vi "Configure LTI ULS.vi"(8 "error in (no error)":errorcluster, 10 "Datalogger Enqueuer":refnum<class "Message Enqueuer.lvclass">, 11 "LTI ULS Actor in":refnum<class "LTI ULS Actor.lvclass">) -> (0 "error out":errorcluster, 3 "LTI ULS Actor out":refnum<class "LTI ULS Actor.lvclass">)   [LabVIEW 2018, in "LTI ULS Actor.lvlib" / "LTI ULS Actor.lvclass"]
uses:
  LTI ULS Actor.lvclass
  C:/Users/dev/Documents/CODE/LabVIEW/microwaveverify/trunk/MWWL Verification/Sensor Actor/Sensor/Sensor.lvclass
  C:/Program Files (x86)/National Instruments/LabVIEW 2018/vi.lib/ActorFramework/Actor/Actor.lvclass
  <vilib>/ActorFramework/Message Enqueuer/Message Enqueuer.lvclass
  LTI ULS Actor.lvclass/LTI ULS Actor.ctl
  <vilib>/ActorFramework/Actor/Actor.lvclass/Actor.ctl
  MWWL Verification/MWWL Verification Messages/Log Event Msg/Log Event Msg.lvclass/Log Event Msg.ctl
  <vilib>/ActorFramework/Message Enqueuer/Message Enqueuer.lvclass/Message Enqueuer.ctl
  <vilib>/ActorFramework/Message Enqueuer/Enqueue.vi
  MWWL Verification/MWWL Verification Messages/Log Event Msg/Log Event Msg.lvclass
  C:/Program Files (x86)/National Instruments/LabVIEW 2018/vi.lib/ActorFramework/Message/Message.lvclass
  <vilib>/Instr/_visa.llb/VISA Configure Serial Port (Instr).vi
  <vilib>/ActorFramework/Message Priority Queue/Priority Enqueue.vi
  Sensor Actor/Sensor/Sensor.lvclass
  <vilib>/ActorFramework/Actor/Actor.lvclass
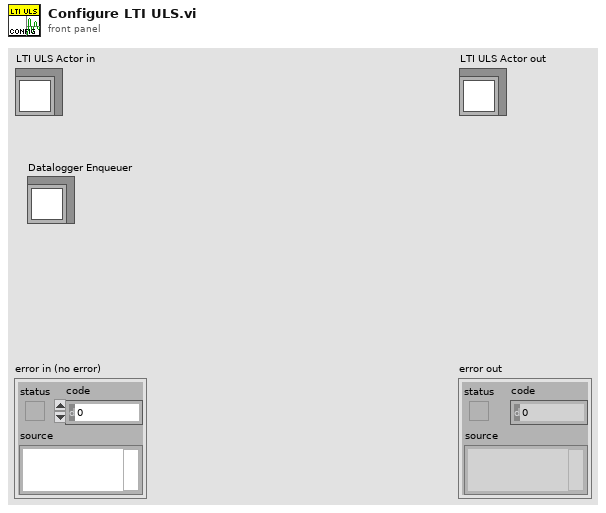
[diagram p1: front panel]
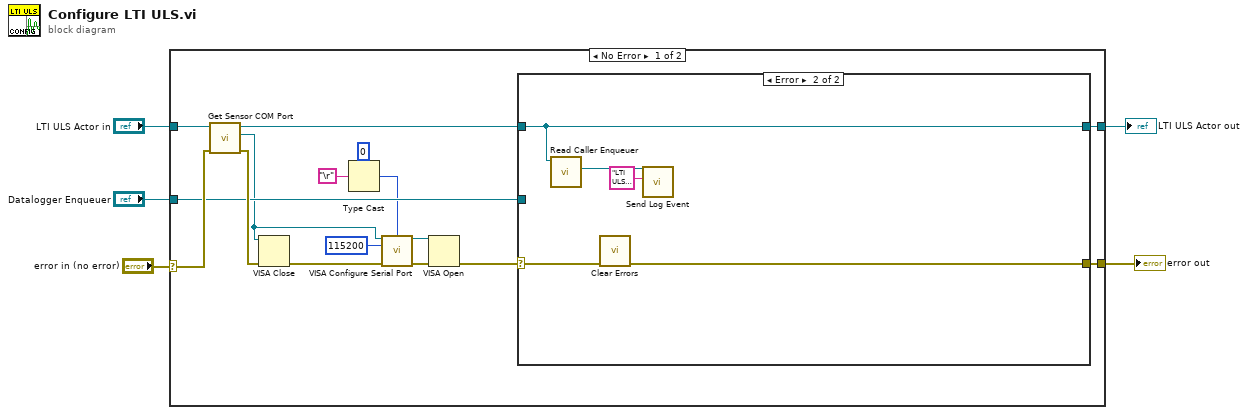
[diagram p0: block diagram]
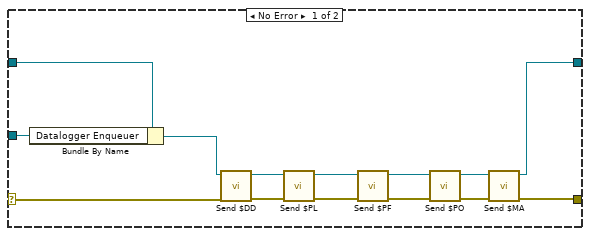
[diagram p2: hidden frame]
diagram:
  n1 = case shown="No Error" "error in (no error)" {
    selector: "error in (no error)" -> [w12 w42]
    tunnel: [w14 w42] -> w4
    tunnel: [w15 w41] -> w2
    tunnel: "LTI ULS Actor in" -> [w21 w41]
    tunnel: "Datalogger Enqueuer" -> [w11 _]
    frame No Error {
      n2 = call "Get Sensor COM Port.vi"("error in (no error)"=w12, "Sensor in"=w21) -> ("error out"=w13:errorcluster, "COM Port"=w9:refnum<visa-resource-name>, "Sensor out"=w16:refnum<class "LTI ULS Actor.lvclass">)  [unwired: 7 in]
      n3 = VISA Close(VISA resource name=w9, error in (no error)=w13) -> (error out=w20:errorcluster)
      n4 = Type Cast(type=u8 0 ("termination char\n(0xA = '\\n' = LF)"), x="\r") -> (*(type *) &x=w7:u8)
      n5 = call-poly "VISA Configure Serial Port"("VISA resource name"=w9, "termination char\n(0xA = '\\n' = LF)"=w7, "baud rate (9600)"=u32 115200, "error in (no error)"=w20) -> ("VISA resource name out"=w18:refnum<visa-resource-name>, "error out"=w19:errorcluster)  [unwired: 10 in]
      n6 = VISA Open(error in (no error)=w19, VISA resource name=w18) -> (error out=w17:errorcluster)  [unwired: 3 in, 1 out]
      n7 = case shown="Error" w17 {
        selector: w17 -> [w33 w38]
        tunnel: w16 -> [w34 w36]
        tunnel: [w25 w36] -> w15
        tunnel: [w26 w37] -> w14
        tunnel: w11 -> [w35 _]
        frame No Error {
          n8 = Bundle By Name(cluster=w34, "Datalogger Enqueuer"=w35) -> (w31:refnum<class "LTI ULS Actor.lvclass">)
          n9 = call "Send $DD.vi"("error in (no error)"=w33, "LTI ULS Actor in"=w31) -> ("error out"=w32:errorcluster, "LTI ULS Actor out"=w30:refnum<class "LTI ULS Actor.lvclass">)  [unwired: 8 in]
          n10 = call "Send $PL.vi"("error in (no error)"=w32, "LTI ULS Actor in"=w30) -> ("error out"=w29:errorcluster, "LTI ULS Actor out"=w22:refnum<class "LTI ULS Actor.lvclass">)  [unwired: 8 in]
          n11 = call "Send $PF.vi"("error in (no error)"=w29, "LTI ULS Actor in"=w22) -> ("error out"=w28:errorcluster, "LTI ULS Actor out"=w23:refnum<class "LTI ULS Actor.lvclass">)  [unwired: 8 in]
          n12 = call "Send $PO.vi"("error in (no error)"=w28, "LTI ULS Actor in"=w23) -> ("error out"=w27:errorcluster, "LTI ULS Actor out"=w24:refnum<class "LTI ULS Actor.lvclass">)  [unwired: 8 in]
          n13 = call "Send $MA.vi"("error in (no error)"=w27, "LTI ULS Actor in"=w24) -> ("error out"=w26:errorcluster, "LTI ULS Actor out"=w25:refnum<class "LTI ULS Actor.lvclass">)  [unwired: 8 in]
        }
        frame Error {
          n14 = call <vilib>:"Read Caller Enqueuer.vi"("Actor"=w36) -> ("Caller Enqueuer"=w40:refnum<class "Message Enqueuer.lvclass">)  [unwired: 10 in]
          n15 = call <vilib>:"Clear Errors.vi"("error in (no error)"=w38) -> ("error out"=w37:errorcluster)  [unwired: 5 in, 1 out]
          n16 = call "Send Log Event.vi"("Event Text"="LTI ULS  Init  Failed.\nAbort and Re-Initialize." ("message"), "Message Enqueuer"=w40) -> ()  [unwired: 8 in, 2 out]
        }
      }
    }
    frame Error {
    }
  }
  "error out" <- w4
  "LTI ULS Actor out" <- w2
